vi "Update Class Icon.vi"(8 "error in (no error)":errorcluster, 9 "UI Icon":refnum<class "Icon.lvclass">, 10 "Icon":refnum<class "Icon.lvclass">, 11 "Rename in":refnum<class "ProjectItem.lvclass">) -> (0 "error out":errorcluster, 3 "Rename out":refnum<class "ProjectItem.lvclass">)   [LabVIEW 2019, in "ProjectItem.lvclass"]
uses:
  ProjectItem.lvclass
  <vilib>/LabVIEW Icon API/lv_icon/Classes/Icon/Icon.lvclass
  ProjectItem.lvclass/ProjectItem.ctl
  <vilib>/LabVIEW Icon API/LabVIEW Icon API.lvlib
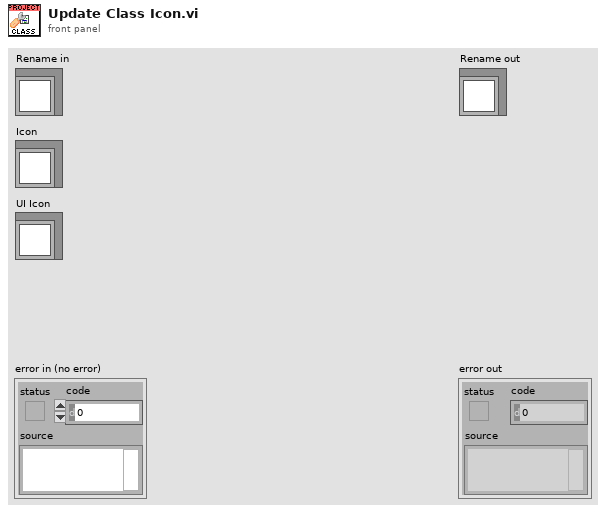
[diagram p1: front panel]
types:
  T1 = cluster{"Class":refnum<vi>, "DynamicVIs":refnum<vi>[], "StaticVIs":refnum<vi>[], "Controls":refnum<vi>[], "Name":string, "Icon":refnum<class "Icon.lvclass">, "Wire Foreground Color":u32}[]
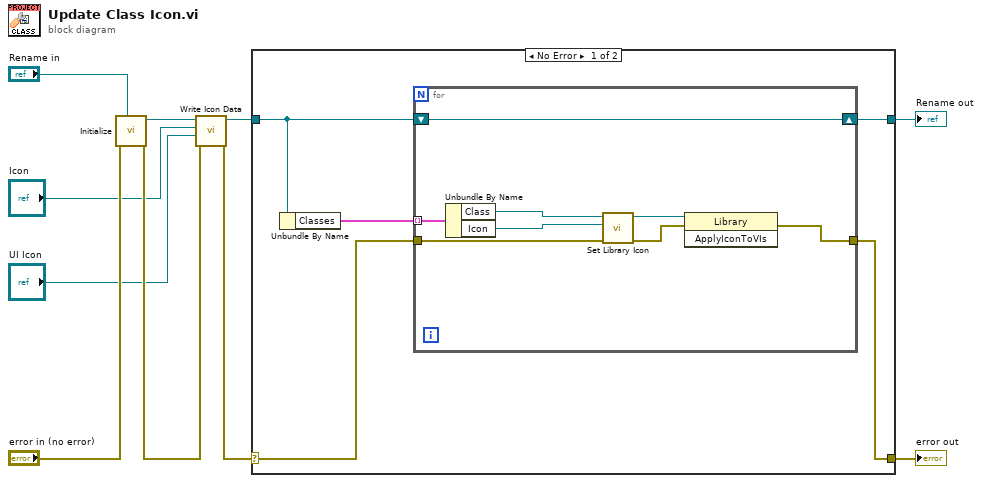
[diagram p0: block diagram]
diagram:
  n1 = call "Initialize.vi"("ProjectItem"="Rename in", "error in (no error)"="error in (no error)") -> ("error out"=w4:errorcluster, "ProjectItem out"=w6:refnum<class "ProjectItem.lvclass">)  [unwired: 8 in]
  n2 = call "Write Icon Data.vi"("error in (no error)"=w4, "UI Icon"="UI Icon", "Icon"="Icon", "ProjectItem in"=w6) -> ("error out"=w3:errorcluster, "ProjectItem out"=w5:refnum<class "ProjectItem.lvclass">)  [unwired: 6 in]
  n3 = case shown="No Error" w3 {
    selector: w3 -> [w11 w25]
    tunnel: [w15 w25] -> w10
    tunnel: [w14 w24] -> w9
    tunnel: w5 -> [w12 w24]
    frame No Error {
      n4 = Unbundle By Name(w12) -> ("Classes"=w13:T1)
      n5 = for {
        tunnel: [w17] -> w15
        tunnel: w13 -> [w23] mode=indexing
        tunnel: w11 -> [w21]
        shift-right: [w20] -> w14
        shift-left: w12 -> [w20]
        n6 = Unbundle By Name(w23) -> ("Class"=w22:refnum<vi>, "Icon"=w16:refnum<class "Icon.lvclass">)
        n7 = call <vilib>:"Set Library Icon.vi"("error in (no error)"=w21, "Icon"=w16, "Library Refnum in"=w22) -> ("error out"=w18:errorcluster, "Library Refnum out"=w19:refnum<vi>)  [unwired: 7 in]
        n8 = invoke class="Library" method="ApplyIconToVIs"(reference=w19, error in=w18) -> (error out=w17:errorcluster)  [unwired: 1 in, 2 out]
      }
    }
    frame Error {
    }
  }
  "error out" <- w10
  "Rename out" <- w9
